vi "linear fit to sensor location.vi"() -> ()   [LabVIEW 2017]
uses:
  <vilib>/Analysis/Matrix/Datatypes/RealMatrix.ctl
  <vilib>/Analysis/Matrix/Datatypes/ComplexMatrix.ctl
  <vilib>/Analysis/7linalg.llb/Eigenvalue and Vectors Output Option.ctl
  <vilib>/Analysis/baseanly.llb/Real A x B.vi
  <vilib>/Analysis/7linalg.llb/Real Eigenvalues and Vectors.vi
  <vilib>/imath/engines/lvmath2/RunTimeEngine/BuiltInFunctions/dot/NIMS_dot(GV,GV).vi
  <instcachedir>/0/NIMS_dot(GV,GV)_B9FAA411F4494E9B94D442721014A3FA.lvgen/NIMS_dot(GV,GV)_B9FAA411F4494E9B94D442721014A3FA_000.vi
  <vilib>/imath/engines/lvmath2/RunTimeEngine/BuiltInFunctions/cross/NIMS_cross(GV,GV).vi
  <instcachedir>/0/NIMS_cross(GV,GV)_40C294A955894C4D81233A182CF84C03.lvgen/NIMS_cross(GV,GV)_40C294A955894C4D81233A182CF84C03_000.vi
  <vilib>/imath/engines/lvmath2/RunTimeEngine/ArithmeticOperatorToken/NIMS_ArithmeticOperator_plus.vi
  <instcachedir>/0/NIMS_ArithmeticOperator_plus_9255C7DA94A9479C92F91DC2DA9A664F.lvgen/NIMS_ArithmeticOperator_plus_9255C7DA94A9479C92F91DC2DA9A664F_004.vi
  <vilib>/imath/engines/lvmath2/RunTimeEngine/ArithmeticOperatorToken/NIMS_ArithmeticOperator_minus.vi
  <instcachedir>/0/NIMS_ArithmeticOperator_minus_0AD0C6F3574E48218C82EC0DAEF38AC8.lvgen/NIMS_ArithmeticOperator_minus_0AD0C6F3574E48218C82EC0DAEF38AC8_003.vi
  <vilib>/imath/engines/lvmath2/RunTimeEngine/ErrorHandling/NIMS_Create Error From Enums.vi
  <vilib>/imathl/engines/lvmath/Functions/Error Handling/Create Error.vi
  <vilib>/imath/engines/lvmath2/RunTimeEngine/NodeEndStatement/NIMS_NodeEndStatement_Output.vi
  <instcachedir>/0/NIMS_NodeEndStatement_Output_53EC0D466D134D7ABD903AC30B43404B.lvgen/NIMS_NodeEndStatement_Output_53EC0D466D134D7ABD903AC30B43404B_005.vi
  <vilib>/imath/engines/lvmath2/RunTimeEngine/ErrorHandling/NIMS_Finalize Error.vi
  <vilib>/imath/engines/lvmath2/RunTimeEngine/ErrorHandling/NIMS_Error From Error Code.vi
  <vilib>/imath/engines/lvmath2/RunTimeEngine/BuiltInFunctions/roots/NIMS_roots.vi
  <instcachedir>/0/NIMS_roots_5371068BAABD481CB00E0B78F1D2DC4F.lvgen/NIMS_roots_5371068BAABD481CB00E0B78F1D2DC4F_000.vi
  <vilib>/imath/engines/lvmath2/RunTimeEngine/BuiltInFunctions/imag/NIMS_imag(Complex).vi
  <instcachedir>/0/NIMS_imag(Complex)_3180D40D00C843A49C2B33397F857BF3.lvgen/NIMS_imag(Complex)_3180D40D00C843A49C2B33397F857BF3_002.vi
  <vilib>/imath/engines/lvmath2/RunTimeEngine/VariableToken/Support/NIMS_Vector Boolean Index to I32 Index.vi
  <vilib>/imath/engines/lvmath2/RunTimeEngine/IndexRead/NIMS V(V).vi
  <instcachedir>/0/NIMS V(V)_298D9CB7BFEB42B8BC8D9C3C28AE8C70.lvgen/NIMS V(V)_298D9CB7BFEB42B8BC8D9C3C28AE8C70_000.vi
  <vilib>/imath/engines/lvmath2/RunTimeEngine/BuiltInFunctions/length/NIMS_length(GV).vi
  <instcachedir>/0/NIMS_length(GV)_08A3D13377FD4E4B96F5795FBF3698FA.lvgen/NIMS_length(GV)_08A3D13377FD4E4B96F5795FBF3698FA_001.vi
  <vilib>/imath/engines/lvmath2/RunTimeEngine/RangeToken/NIMS_Range_R2 - Integer.vi
  <instcachedir>/0/NIMS_Range_R2 - Integer_B2C3C6B11D0E4F789E1772ACB483EB02.lvgen/NIMS_Range_R2 - Integer_B2C3C6B11D0E4F789E1772ACB483EB02_000.vi
  <vilib>/imath/engines/lvmath2/RunTimeEngine/CommandStatement/MC_CommandStatement_break.vi
  <vilib>/imath/engines/lvmath2/RunTimeEngine/VariableToken/NIMS_VariableToken_CondDefinedDefinedByReplace.vi
  <instcachedir>/0/NIMS_VariableToken_CondDefinedDefinedByReplace_D162CFFC24174562A9FEA619A91E1A56.lvgen/NIMS_VariableToken_CondDefinedDefinedByReplace_D162CFFC24174562A9FEA619A91E1A56_000.vi
  <vilib>/imath/engines/lvmath2/RunTimeEngine/IndexRead/NIMS V(S).vi
  <instcachedir>/0/NIMS V(S)_0488751826AF41519A22953C041130DC.lvgen/NIMS V(S)_0488751826AF41519A22953C041130DC_003.vi
  <vilib>/imath/engines/lvmath2/RunTimeEngine/ArithmeticOperatorToken/NIMS_ArithmeticOperator_power(S).vi
  <instcachedir>/0/NIMS_ArithmeticOperator_power(S)_86B1D76B77564424912EAFCCCC7488ED.lvgen/NIMS_ArithmeticOperator_power(S)_86B1D76B77564424912EAFCCCC7488ED_010.vi
  <instcachedir>/0/NIMS_ArithmeticOperator_plus_9255C7DA94A9479C92F91DC2DA9A664F.lvgen/NIMS_ArithmeticOperator_plus_9255C7DA94A9479C92F91DC2DA9A664F_001.vi
  <instcachedir>/0/NIMS_ArithmeticOperator_plus_9255C7DA94A9479C92F91DC2DA9A664F.lvgen/NIMS_ArithmeticOperator_plus_9255C7DA94A9479C92F91DC2DA9A664F_000.vi
  <instcachedir>/0/NIMS_ArithmeticOperator_power(S)_86B1D76B77564424912EAFCCCC7488ED.lvgen/NIMS_ArithmeticOperator_power(S)_86B1D76B77564424912EAFCCCC7488ED_011.vi
  <vilib>/imath/engines/lvmath2/RunTimeEngine/BuiltInFunctions/sum/NIMS_sum(GV).vi
  <instcachedir>/0/NIMS_sum(GV)_67F5EC36BC034E54A6BEC5B0673C00E5.lvgen/NIMS_sum(GV)_67F5EC36BC034E54A6BEC5B0673C00E5_001.vi
  <vilib>/imath/engines/lvmath2/RunTimeEngine/IndexReplace/NIMS V(S)=S.vi
  <instcachedir>/0/NIMS V(S)=S_3F4D177D41884A9C969E5FA0B22E4B28.lvgen/NIMS V(S)=S_3F4D177D41884A9C969E5FA0B22E4B28_001.vi
  <vilib>/imath/engines/lvmath2/RunTimeEngine/VariableToken/NIMS_VariableToken_CondDefined.vi
  <instcachedir>/0/NIMS_VariableToken_CondDefined_6E7F1EE7F80E48298C84CF05BD736261.lvgen/NIMS_VariableToken_CondDefined_6E7F1EE7F80E48298C84CF05BD736261_000.vi
  <vilib>/imath/engines/lvmath2/RunTimeEngine/BuiltInFunctions/min/1 input/NIMS_min(CV).vi
  <instcachedir>/0/NIMS_min(CV)_524FAF52DF2F460EB3AC993C19173CA1.lvgen/NIMS_min(CV)_524FAF52DF2F460EB3AC993C19173CA1_000.vi
  <vilib>/imath/engines/lvmath/Functions/Error Handling/MergeErrorsWrapper.vi
  <instcachedir>/0/NIMS_NodeEndStatement_Output_53EC0D466D134D7ABD903AC30B43404B.lvgen/NIMS_NodeEndStatement_Output_53EC0D466D134D7ABD903AC30B43404B_000.vi
  <instcachedir>/0/NIMS_NodeEndStatement_Output_53EC0D466D134D7ABD903AC30B43404B.lvgen/NIMS_NodeEndStatement_Output_53EC0D466D134D7ABD903AC30B43404B_001.vi
  <vilib>/Analysis/NI_AALPro.lvlib
  <vilib>/Analysis/NI_AALBase.lvlib
  <vilib>/Analysis/Matrix/NI_Matrix.lvlib
panel:
  out "v":cdb[](array[numeric])
  out "allt":cdb[](array[numeric])
  out "magnet position":dbl[](array[numeric])
  out "t":dbl
  out "H":dbl[](array[numeric])
  out "r":dbl[](array[numeric])
  out "min index(es)":i32
  out "Eigenvectors":T1
  out "Eigenvalues":cdb[](array[numeric])
  out "R":T2
  in  "B-field":T2=[[1053.13, -732.23, 1552.64], [92.19, -296.58, -283.3], [-780.76, 344.14, 683.59], [408.5, -47.07, 22.36], [24.32, -1008.69, 2363.28], [558.11, -273.73, 89.84], [956.74, 360.64, 1571.88], [238.87, -684.08, -167.48]]
  in  "Sensor locations":T2=[[0.0, 0.0, 0.0], [0.0, 75.0, 0.0], [64.951, -37.5, 0.0], [-64.951, -37.5, 0.0], [25.0, 0.0, 0.0], [-50.0, 0.0, 0.0], [0.0, -25.0, 0.0], [0.0, 50.0, 0.0]]
  # "X: 1053.13 92.19 -780.76 408.50 24.32 558.11 956.74 238.87  \nY: -732.23 -296.58 344.14 -47.07 -1008.69 -273.73 360.64 -684.08  \nZ: 1552.64 -283.30 683.59 22.36 2363.28 89.84 1571.88 -167.48"
  # "X: 1053.13 92.19 -780.76 408.50 24.32 558.11 956.74 238.87  \nY: -732.23 -296.58 344.14 -47.07 -1008.69 -273.73 360.64 -684.08  \nZ: 1552.64 -283.30 683.59 22.36 2363.28 89.84 1571.88 -167.48"
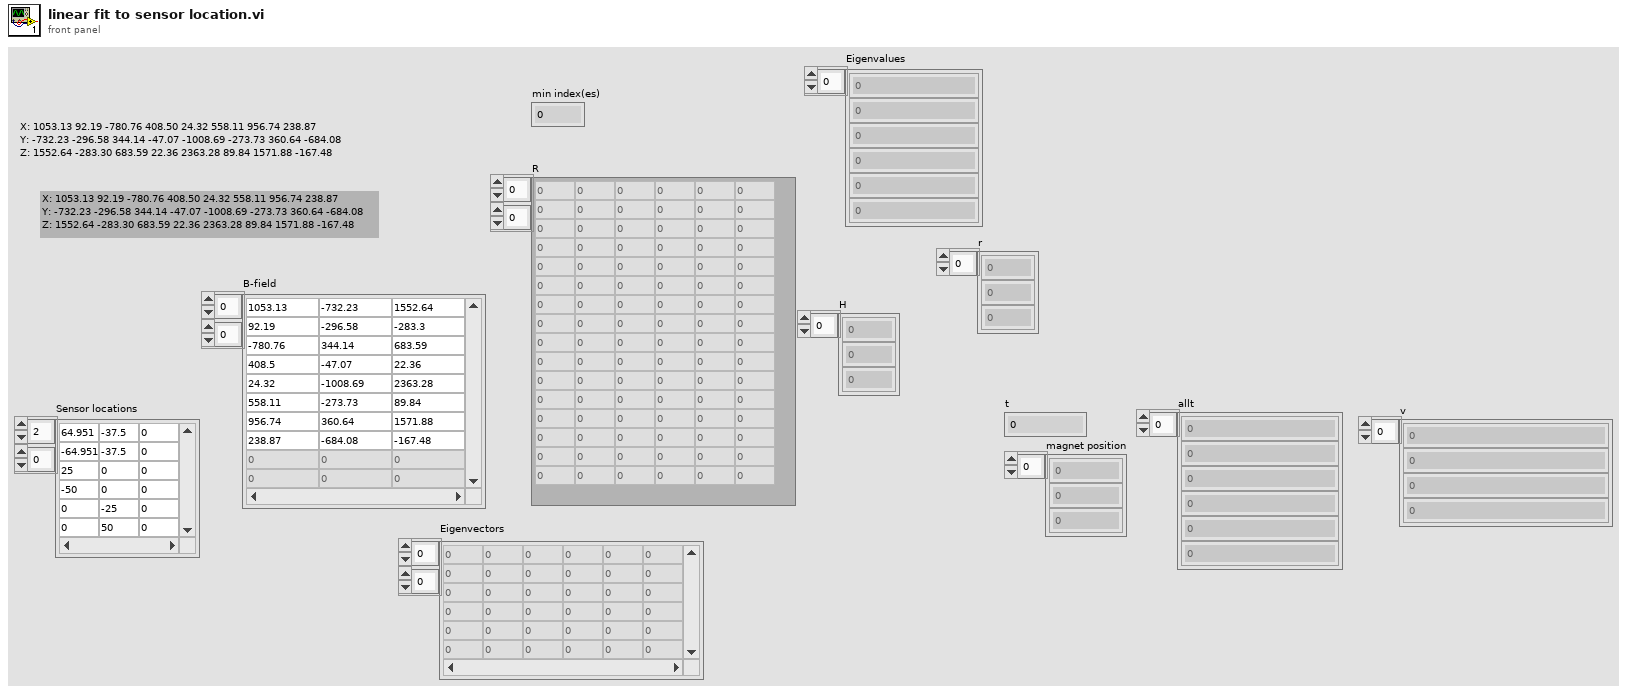
[diagram p1: front panel]
types:
  T1 = typedef "NI_Matrix.lvlib/ComplexMatrix.ctl" = cdb[][]
  T2 = typedef "NI_Matrix.lvlib/RealMatrix.ctl" = dbl[][]
  T3 = typedef "NI_AALPro.lvlib/Eigenvalue and Vectors Output Option.ctl" = i32
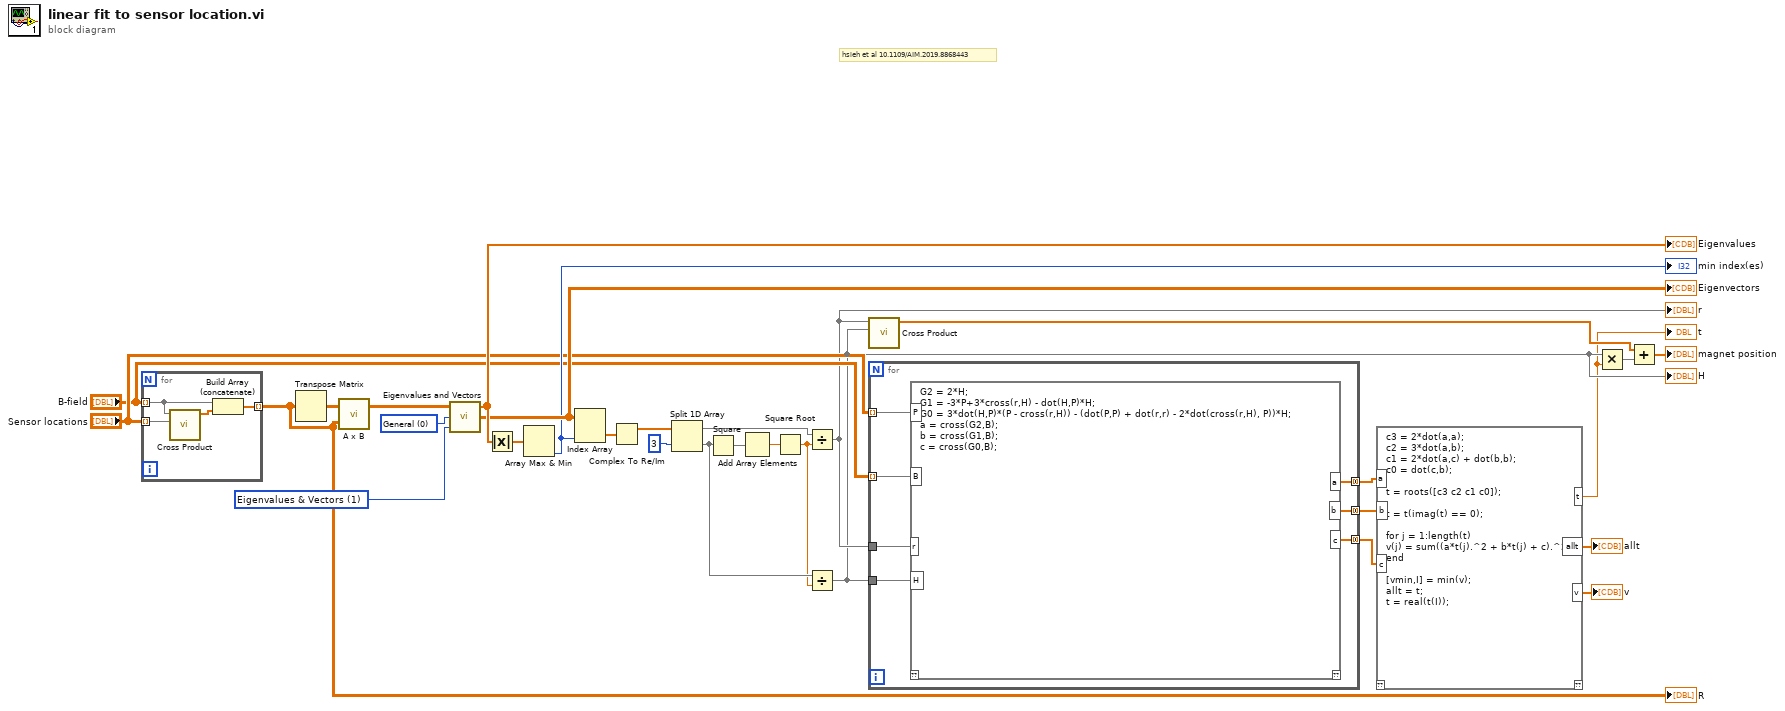
[diagram p0: block diagram]
diagram:
  w25 = T3 1 items=["Eigenvalues", "Eigenvalues & Vectors"] ("output option")
  w26 = 0 items=["General", "Symmetric"] ("matrix type")
  # "hsieh et al 10.1109/AIM.2019.8868443"
  n1 = for {
    tunnel: "B-field" -> [w31] mode=indexing
    tunnel: "Sensor locations" -> [w34] mode=indexing
    tunnel: [w32] -> w21 mode=indexing
    n2 = call <vilib>:"Cross Product.vi"("B Vector"=w34, "A Vector"=w31) -> ("Cross Product"=w33:dbl[])  [unwired: 8 in, 1 out]
    n3 = Build Array (concatenate)(w31, w33) -> (w32:dbl[])
  }
  "R" <- w21
  n4 = Transpose Matrix(1:w21) -> (0:w30:dbl[][])
  n5 = call-poly <vilib>:"A x B.vi"("B"=w21, "A"=w30) -> ("A x B"=w29:T2)  [unwired: 1 out]
  n6 = call-poly <vilib>:"Eigenvalues and Vectors.vi"("output option"=w25, "matrix type"=w26, "Input Matrix"=w29) -> ("Eigenvectors"=w23:T1, "Eigenvalues"=w28:cdb[])  [unwired: 1 out]
  "Eigenvalues" <- w28
  "Eigenvectors" <- w23
  n7 = Absolute Value(x=w28) -> (abs(x)=w27:dbl[])
  n8 = Array Max & Min(array=w27) -> (min index (indices)=w22:i32)  [unwired: 3 out]
  "min index(es)" <- w22
  n9 = Index Array(array=w23, index (col)=w22) -> (element=w24:cdb[])  [unwired: 1 in]
  n10 = Complex To Re/Im(x + iy=w24) -> (x=w20:dbl[])  [unwired: 1 out]
  n11 = Split 1D Array(array=w20, index=3) -> (first subarray=w16:dbl[], second subarray=w15:dbl[])
  n12 = Square(x=w15) -> (x^2=w17:dbl[])
  n13 = Add Array Elements(numeric array=w17) -> (sum=w18:dbl)
  n14 = Square Root(x=w18) -> (sqrt(x)=w14:dbl)
  n15 = Divide(x=w16, y=w14) -> (x/y=w8:dbl[])
  "r" <- w8
  n16 = Divide(x=w15, y=w14) -> (x/y=w6:dbl[])
  "H" <- w6
  n17 = call <vilib>:"Cross Product.vi"("B Vector"=w6, "A Vector"=w8) -> ("Cross Product"=w7:dbl[])  [unwired: 8 in, 1 out]
  n18 = for {
    tunnel: "Sensor locations" -> [w41] mode=indexing
    tunnel: "B-field" -> [w40] mode=indexing
    tunnel: w8 -> [w39]
    tunnel: w6 -> [w38]
    tunnel: [w37] -> w11 mode=concatenating
    tunnel: [w36] -> w10 mode=concatenating
    tunnel: [w35] -> w9 mode=concatenating
    n19 = mathscript code="G2 = 2*H;\nG1 = -3*P+3*cross(r,H) - dot(H,P)*H;\nG0 = 3*dot(H,P)*(P - cross(r,H)) - (dot(P,P) + dot(r,r) - 2*dot(cross(r,H), P))*H;\na = cross(G2,B);\nb = cross(G1,B);\nc = cross(G0,B);"("P"=w41, "B"=w40, "r"=w39, "H"=w38) -> ("a"=w37:dbl[], "b"=w36:dbl[], "c"=w35:dbl[])  [unwired: 1 in, 1 out]
  }
  n20 = mathscript code="c3 = 2*dot(a,a);\nc2 = 3*dot(a,b);\nc1 = 2*dot(a,c) + dot(b,b);\nc0 = dot(c,b);\n\nt = roots([c3 c2 c1 c0]);\n\nt = t(imag(t) == 0);\n\nfor j = 1:length(t)\nv(j) = sum((a*t(j).^2 + b*t(j) + c).^2);\nend\n\n[vmin,I] = min(v);\nallt = t;\nt = real(t(I));"("a"=w11, "b"=w10, "c"=w9) -> ("t"=w5:dbl, "allt"=→"allt":cdb[], "v"=→"v":cdb[])  [unwired: 1 in, 1 out]
  "t" <- w5
  n21 = Multiply(x=w6, y=w5) -> (x*y=w4:dbl[])
  n22 = Add(x=w7, y=w4) -> (x+y=→"magnet position":dbl[])
